vi "ProcessData.vi"(8 "error in (no error)":errorcluster, 9 "State":T1, 10 "Analog Data":T3, 11 "BehaviorClassification in":refnum<class "ClassDiscrimination.lvclass">) -> (0 "error out":errorcluster, 1 "Fixated":bool, 2 "Trigger":T2=enum."Broke Fixation", 3 "BehaviorClassification out":refnum<class "ClassDiscrimination.lvclass">)   [LabVIEW 2010, in "ClassDiscrimination.lvclass"]
uses:
  ClassDiscrimination.lvclass
  Core SubVIs/Controls/TYPE - Analog Data.ctl
  Trial Based Experiment.lvsc/Trigger.ctl
  Trial Based Experiment.lvsc/State.ctl
  ClassDiscrimination.lvclass/ClassDiscrimination.ctl
  <vilib>/measure/madcrms.llb/Basic Averaged DC-RMS for 1 Chan.vi
  Trial Based Experiment.lvsc
  Core SubVIs/Core SubVIs.lvlib
  <vilib>/measure/NI_MAPro.lvlib
  Acquisition/BehaviorData/BehaviorData.lvclass
panel:
  in  "Adjustment Rate":dbl=0.002
  in  "Target Distance":dbl=300.0
  in  "Incorrect":bool
  in  "Correct":bool
  in  "Toggle Fixation":bool
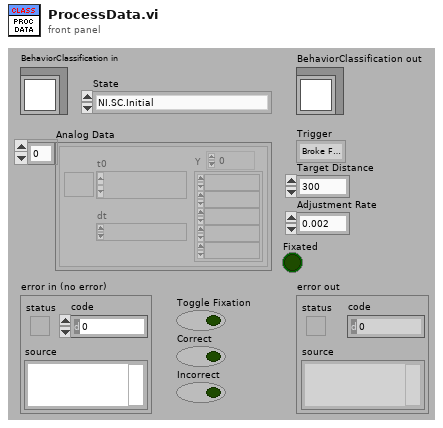
[diagram p1: front panel]
types:
  T1 = typedef "Trial Based Experiment.lvsc/State.ctl" = enum16{"NI.SC.Initial", "NI.SC.History", "NI.SC.ShallowHistory", "NI.SC.Terminal", "Cleanup", "State", "State\\Region\\Pause", "State\\Region\\Response Period", "State\\Region\\Delay Period", "State\\Region\\Hold Fixation", "State\\Region\\Acquire Fixation", "State\\Region\\Abort Trial", "State\\Region\\End Trial", "State\\Region\\Intertrial", "State\\Region\\Start Trial"}
  T2 = typedef "Trial Based Experiment.lvsc/Trigger.ctl" = enum16{"NULL", "Fixated", "Broke Fixation", "Stop", "Correct Response", "Incorrect Response", "Timeout"}
  T3 = typedef "Core SubVIs.lvlib/TYPE - Analog Data.ctl" = waveform(dbl)[]
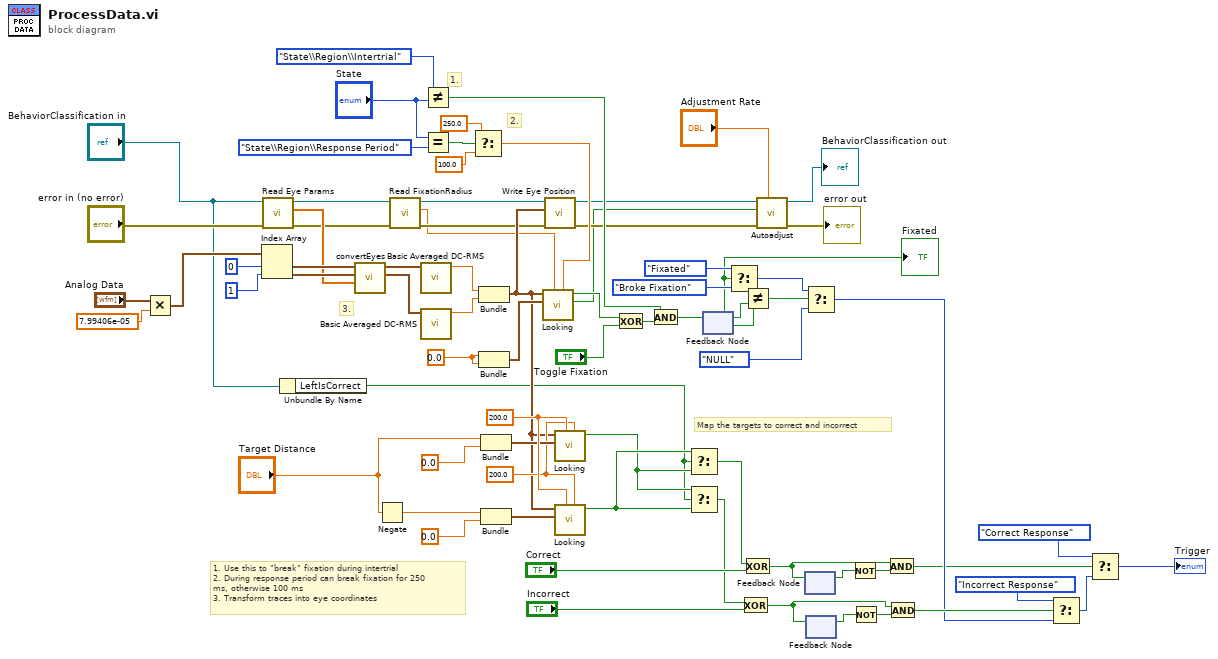
[diagram p0: block diagram]
diagram:
  w35 = 200.0
  w44 = 200.0 ("Fixation Radius (px)")
  w49 = 0.0
  # "3."
  # "1."
  # "2."
  # "1. Use this to \"break\" fixation during intertrial\n2. During response period can break fixation for 250\nms, otherwise 100 ms\n3. Transform traces into eye coordinates"
  # "Map the targets to correct and incorrect"
  n1 = Multiply(x="Analog Data", y=7.99406e-05) -> (x*y=w10:T3)
  n2 = Index Array(array=w10, index #1=0 ("index"), index #2=1 ("index")) -> (element #1=w73:waveform(dbl), element #2=w72:waveform(dbl))
  n3 = call-dynamic "Read Eye Params.vi"("error in (no error)"="error in (no error)", "TrialBasedExperiment in"="BehaviorClassification in") -> ("error out"=w26:errorcluster, "Eye Params"=w64:dbl[], "TrialBasedExperiment out"=w27:refnum<class "ClassDiscrimination.lvclass">)  [unwired: 7 in]
  n4 = Unbundle By Name("BehaviorClassification in") -> ("LeftIsCorrect"=w22:bool)
  n5 = call "convertEyes.vi"("Params"=w64, "Vertical"=w72, "Horizontal"=w73) -> ("Vertical Calibrated"=w70:waveform(dbl), "Horizontal Calibrated"=w71:waveform(dbl))  [unwired: 7 in]
  n6 = Negate(x="Target Distance") -> (-x=w29:dbl)
  n7 = call-dynamic "Read FixationRadius.vi"("error in (no error)"=w26, "MatlabExperiment in"=w27) -> ("error out"=w24:errorcluster, "FixationRadius"=w23:dbl, "MatlabExperiment out"=w25:refnum<class "ClassDiscrimination.lvclass">)  [unwired: 7 in]
  n8 = call-poly <vilib>:"Basic Averaged DC-RMS.vi"("signal in"=w71) -> ("DC value"=w52:dbl)  [unwired: 7 in, 3 out]
  n9 = call-poly <vilib>:"Basic Averaged DC-RMS.vi"("signal in"=w70) -> ("DC value"=w51:dbl)  [unwired: 7 in, 3 out]
  n10 = Not Equal?(x=State."State\\Region\\Intertrial", y="State") -> (x != y?=w19:bool)
  n11 = Equal?(x="State", y=State."State\\Region\\Response Period") -> (x = y?=w16:bool)
  n12 = Select(t=250.0 ("Break Timeout (ms)"), s=w16, f=100.0) -> (s? t:f=w13:dbl)
  n13 = Bundle("DC value"=w52, "DC value"=w51) -> (w28:cluster{"DC value":dbl, "DC value":dbl})  [unwired: 1 in]
  n14 = Bundle(w49, w49) -> (w50:cluster{dbl, dbl})  [unwired: 1 in]
  n15 = Bundle("Target Distance"="Target Distance", 0.0) -> (w42:cluster{"Target Distance":dbl, dbl})  [unwired: 1 in]
  n16 = Bundle(w29, 0.0) -> (w40:cluster{dbl, dbl})  [unwired: 1 in]
  n17 = call "Looking.vi"("Break Timeout (ms)"=w13, "Fixation Radius (px)"=w23, "Desired Position"=w50, "Eye Position"=w28) -> ("Looking Unfiltered"=w1:bool, "Looking"=w47:bool)  [unwired: 6 in]
  n18 = call-dynamic "Write Eye Position.vi"("error in (no error)"=w24, "Eye Position"=w28, "TrialBasedExperiment in"=w25) -> ("error out"=w6:errorcluster, "TrialBasedExperiment out"=w7:refnum<class "ClassDiscrimination.lvclass">)  [unwired: 7 in]
  n19 = call "Looking.vi"("Break Timeout (ms)"=w35, "Fixation Radius (px)"=w44, "Desired Position"=w42, "Eye Position"=w28) -> ("Looking"=w33:bool)  [unwired: 6 in, 1 out]
  n20 = call "Looking.vi"("Break Timeout (ms)"=w35, "Fixation Radius (px)"=w44, "Desired Position"=w40, "Eye Position"=w28) -> ("Looking"=w34:bool)  [unwired: 6 in, 1 out]
  n21 = Exclusive Or(1:"Toggle Fixation", 2:w47) -> (0:w20:bool)
  n22 = And(x=w19, y=w20) -> (x .and. y?=w4:bool)
  "Fixated" <- w4
  n23 = Select(t=w34, s=w22, f=w33) -> (s? t:f=w32:bool)
  n24 = Select(t=w33, s=w22, f=w34) -> (s? t:f=w31:bool)
  n25 = feedback #1() -> (w69:bool)  [unwired: 1 in]
  n26 = feedback-in #1(w4) -> ()
  n27 = Select(t=Trigger."Fixated" ("Trigger"), s=w4, f=Trigger."Broke Fixation" ("Trigger")) -> (s? t:f=w67:T2)
  n28 = Exclusive Or(1:"Incorrect", 2:w31) -> (0:w36:bool)
  n29 = Not Equal?(x=w4, y=w69) -> (x != y?=w8:bool)
  n30 = Exclusive Or(1:"Correct", 2:w32) -> (0:w38:bool)
  n31 = call-dynamic "Autoadjust.vi"("Adjustment Rate"="Adjustment Rate", "error in (no error)"=w6, "Fixated"=w1, "TrialBasedExperiment in"=w7) -> ("error out"=→"error out":errorcluster, "TrialBasedExperiment out"=→"BehaviorClassification out":refnum<class "ClassDiscrimination.lvclass">)  [unwired: 6 in]
  n32 = feedback #2() -> (w62:bool)  [unwired: 1 in]
  n33 = feedback-in #2(w38) -> ()
  n34 = Select(t=w67, s=w8, f=Trigger."NULL" ("Trigger")) -> (s? t:f=w57:T2)
  n35 = feedback #3() -> (w60:bool)  [unwired: 1 in]
  n36 = feedback-in #3(w36) -> ()
  n37 = Not(x=w62) -> (.not. x?=w61:bool)
  n38 = Not(x=w60) -> (.not. x?=w59:bool)
  n39 = And(x=w38, y=w61) -> (x .and. y?=w56:bool)
  n40 = And(x=w36, y=w59) -> (x .and. y?=w58:bool)
  n41 = Select(t=Trigger."Incorrect Response", s=w58, f=w57) -> (s? t:f=w55:T2)
  n42 = Select(t=Trigger."Correct Response", s=w56, f=w55) -> (s? t:f=→"Trigger":T2)
